vi "PH_HamamatsuCamera.set Trigger.vi"(0 "i ref in":refnum<vi>, 1 "Cam Handle in":i32, 2 "Trigger Parameters":T1={"Mode"=1, "Polarity"=1, "Times"=1, "Delay"=0.0} {"Polarity" items=["Negative"=1, "Positive"=2]; "Mode" items=["Internal"=1, "External Edge"=2, "External Level"=4, "Software"=32, "Fast Repetition"=64, "TDI"=128, "Trigger Start"=512, "Sync Readout"=1024]}, 4 "Cam Error in":errorcluster, 5 "error in (no error)":errorcluster) -> (14 "i ref out":refnum<vi>, 15 "Cam Handle out":i32, 18 "Cam Error out":errorcluster, 19 "error out":errorcluster)   [LabVIEW 2014, in "PH_HamamatsuCamera.lvlib"]
doc: "This VI sets the trigger parameters of a cam."
uses:
  PH_HamamatsuCamera.lvlib
  PH_Common/PH_Common.lvlib
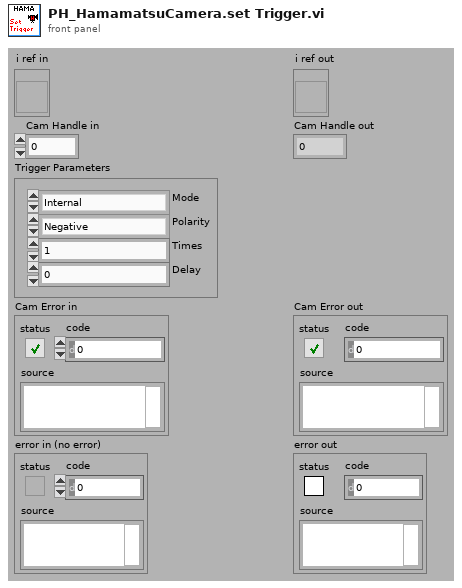
[diagram p1: front panel]
types:
  T1 = cluster{"Mode":u32, "Polarity":u32, "Times":u32, "Delay":dbl}
  T2 = typedef "PH_HamamatsuCamera.lvlib/PH_HamamatsuCamera.i attribute.ctl" = cluster{"Gui Refs":cluster{"Camera Details":refnum<vi>, "ROI":refnum<vi>, "Set ROI to Maximum":refnum<vi>, "Trigger Parameters":refnum<vi>, "Brightness":refnum<vi>, "Shutter":refnum<vi>, "Gain":refnum<vi>, "Trigger Timeout":refnum<vi>, "Trigger Polarity":refnum<vi>, "Trigger Mode":refnum<vi>, "Parameters":refnum<vi>, "Set Cam Parameter":refnum<vi>, "Parameter to set":refnum<vi>, "Value to set":refnum<vi>}, "Cam":cluster{"Handle":i32, "Details":cluster{"Model":string, "Camera ID":string, "Firmware":string}, "Buffer Info":cluster{"height":u32, "width":u32, "datatype":u32}}, "H Offset":cluster{"Value":i32, "Minimum":i32, "Maximum":i32, "Increment":i32}, "V Offset":cluster{"Value":i32, "Minimum":i32, "Maximum":i32, "Increment":i32}, "H Width":cluster{"Value":i32, "Minimum":i32, "Maximum":i32, "Increment":i32}, "V Width":cluster{"Value":i32, "Minimum":i32, "Maximum":i32, "Increment":i32}, "Trigger Parameters":T3, "Trigger Timeout":u32, "Parameters":T4[], "Indicees Cam Parameters":cluster{"Brightness":i32, "Shutter":i32, "Gain":i32}, "Wanted Values":cluster{"Trigger Settings":T3[], "ROI":T5[], "Parameter":cluster{"Name":string, "Value":dbl}[]}}
  T3 = typedef "PH_HamamatsuCamera.lvlib/PH_HamamatsuCamera.Trigger Parameter.ctl" = cluster{"Mode":u32, "Polarity":u32, "Times":u32, "Delay":dbl}
  T4 = typedef "PH_HamamatsuCamera.lvlib/PH_HamamatsuCamera.Parameter Set.ctl" = cluster{"Parameter":string, "Value":dbl, "Writable":bool, "Range":cluster{"min":dbl, "max":dbl, "step":dbl}, "Default":dbl, "Value Names":cluster{"Name":string, "Value":dbl}[], "Text Values":bool}
  T5 = typedef "PH_HamamatsuCamera.lvlib/PH_HamamatsuCamera.ROI.ctl" = cluster{"Horizontal Offset":i32, "Vertical Offset":i32, "Horizontal Width":i32, "Vertical Width":i32}
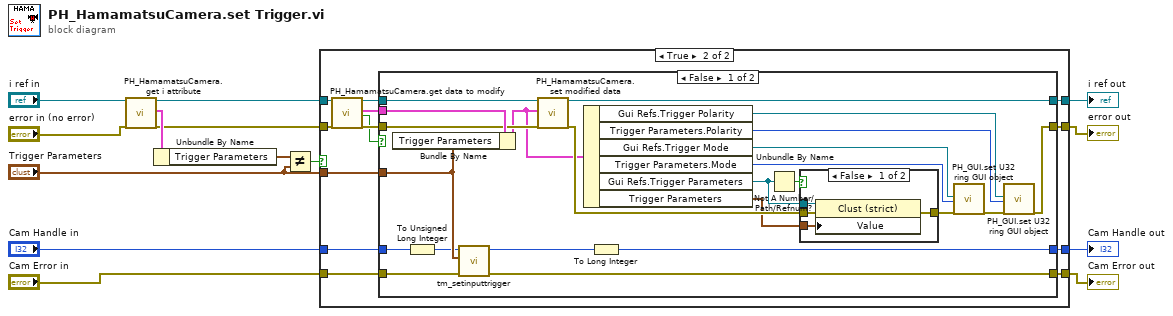
[diagram p0: block diagram]
diagram:
  n1 = call "PH_HamamatsuCamera.get i attribute.vi"("i ref in"="i ref in", "error in (no error)"="error in (no error)") -> ("i ref out"=w8:refnum<vi>, "i attribute"=w12:T2, "error out"=w6:errorcluster)  [unwired: 15 in]
  n2 = Unbundle By Name(w12) -> ("Trigger Parameters"=w9:T3)
  n3 = Not Equal?(x=w9, y="Trigger Parameters") -> (x != y?=w3:bool)
  n4 = case shown="True" w3 {
    tunnel: [w18 w24] -> w11
    tunnel: [w17 w23] -> w10
    tunnel: w8 -> [w18 w30]
    tunnel: "Trigger Parameters" -> [_ w27]
    tunnel: w6 -> [w17 w25]
    tunnel: "Cam Handle in" -> [w16 w22]
    tunnel: "Cam Error in" -> [w15 w21]
    tunnel: [w15 w20] -> w1
    tunnel: [w16 w19] -> w2
    frame False {
    }
    frame True {
      n5 = call "PH_HamamatsuCamera.get data to modify.vi"("i ref in"=w30, "error in (no error)"=w25) -> ("i ref out"=w29:refnum<vi>, "i attribute"=w28:T2, "timed out"=w26:bool, "error out"=w31:errorcluster)  [unwired: 14 in]
      n6 = case shown="False" w26 {
        tunnel: [w35 w62] -> w23
        tunnel: w31 -> [w48 w62]
        tunnel: w29 -> [w54 w63]
        tunnel: w28 -> [w53 _]
        tunnel: [w36 w63] -> w24
        tunnel: w27 -> [w52 _]
        tunnel: w22 -> [w51 w61]
        tunnel: w21 -> [w37 w60]
        tunnel: [w34 w60] -> w20
        tunnel: [w32 w61] -> w19
        frame False {
          n7 = Bundle By Name(cluster=w53, "Trigger Parameters"=w52) -> (w46:T2)
          n8 = To Unsigned Long Integer(number=w51) -> (unsigned 32bit integer=w50:u32)
          n9 = call <userlib>:"tm_setinputtrigger.vi"("error in (no error)"=w37, "Parameters"=w52, "Handle in"=w50) -> ("error out"=w34:errorcluster, "Handle out"=w33:u32)  [unwired: 7 in]
          n10 = call "PH_HamamatsuCamera.set modified data.vi"("i ref in"=w54, "i attribute"=w46, "error in (no error)"=w48) -> ("i ref out"=w36:refnum<vi>, "error out"=w47:errorcluster)  [unwired: 15 in]
          n11 = Unbundle By Name(w46) -> ("Gui Refs.Trigger Polarity"=w41:refnum<vi>, "Trigger Parameters.Polarity"=w39:u32, "Gui Refs.Trigger Mode"=w40:refnum<vi>, "Trigger Parameters.Mode"=w38:u32, "Gui Refs.Trigger Parameters"=w45:refnum<vi>, "Trigger Parameters"=w44:T3)
          n12 = To Long Integer(number=w33) -> (32bit integer=w32:i32)
          n13 = Not A Number/Path/Refnum?(number/path/refnum=w45) -> (NaN/Path/Refnum?=w49:bool)
          n14 = case shown="False" w49 {
            tunnel: w47 -> [w58 w59]
            tunnel: [w57 w59] -> w42
            tunnel: w45 -> [w56 _]
            tunnel: w44 -> [w55 _]
            frame False {
              n15 = property class="Clust (strict)"(reference=w56, error in=w58, "Value"=w55) -> (error out=w57:errorcluster)  [unwired: 1 out]
            }
            frame True {
            }
          }
          n16 = call "PH_GUI.set U32 ring GUI object.vi"("Ring Ref"=w40, "Value"=w38, "error in (no error)"=w42) -> ("error out"=w43:errorcluster)  [unwired: 16 in]
          n17 = call "PH_GUI.set U32 ring GUI object.vi"("Ring Ref"=w41, "Value"=w39, "error in (no error)"=w43) -> ("error out"=w35:errorcluster)  [unwired: 16 in]
        }
        frame True {
        }
      }
    }
  }
  "error out" <- w10
  "i ref out" <- w11
  "Cam Handle out" <- w2
  "Cam Error out" <- w1
